vi "Read Single Digital.vi"(0 "Device ID":T3(ring), 5 "Module":T2(ring), 7 "Digital_Input":T1(ring), 11 "error in":errorcluster) -> (4 "Device ID Out":T3(ring), 6 "Value":bool, 15 "error out":errorcluster)   [LabVIEW 2010]
doc: "This VI reads a single digital input from the transfer area."
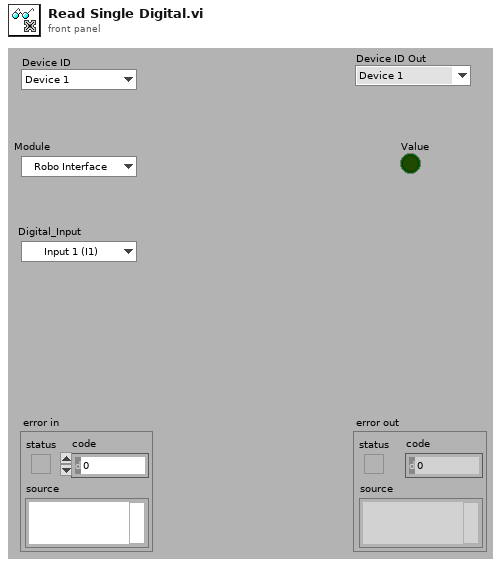
[diagram p1: front panel]
types:
  T1 = enum8{"Input 1 (I1)", "Input 2 (I2)", "Input 3 (I3)", "Input 4 (I4)", "Input 5 (I5)", "Input 6 (I6)", "Input 7 (I7)", "Input 8 (I8)"}
  T2 = enum8{"Robo Interface", "Extension 1", "Extension 2", "Extension 3"}
  T3 = enum16{"Device 1", "Device 2", "Device 3", "Device 4", "Device 5", "Device 6", "Device 7", "Device 8"}
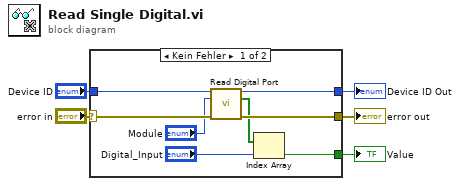
[diagram p0: block diagram]
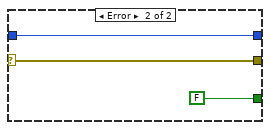
[diagram p2: hidden frame]
diagram:
  n1 = case shown="Kein Fehler" "error in" {
    selector: "error in" -> [w10 w16]
    tunnel: [w9 w16] -> w4
    tunnel: "Device ID" -> [w12 w15]
    tunnel: [w11 w15] -> w2
    tunnel: [w6 FALSE] -> w1
    frame No Error {
      n2 = call "Read Digital Port.vi"("Device ID"=w12, "Module"="Module", "error in"=w10) -> ("Device ID Out"=w11:T3, "Value"=w8:bool[], "error out"=w9:errorcluster)  [unwired: 10 out]
      n3 = Index Array(array=w8, index="Digital_Input") -> (element=w6:bool)
    }
    frame Error {
    }
  }
  "error out" <- w4
  "Device ID Out" <- w2
  "Value" <- w1
